vi "Close.vi"(8 "error in":errorcluster, 11 "Comport":refnum<visa-resource-name>) -> (0 "error out":errorcluster)   [LabVIEW 2020, in "MicroPythonClient.lvlib"]
doc: "Closes the comport to the target"
uses:
  MicroPythonClient.lvlib
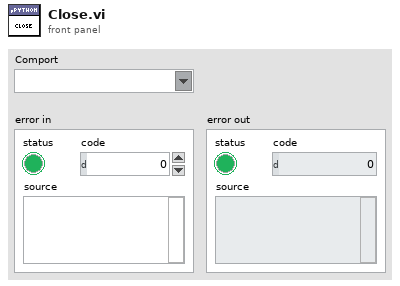
[diagram p1: front panel]
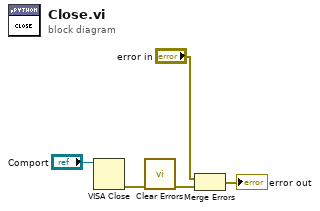
[diagram p0: block diagram]
diagram:
  n1 = VISA Close(VISA resource name="Comport") -> (error out=w2:errorcluster)  [unwired: 1 in]
  n2 = call <vilib>:"Clear Errors.vi"("error in (no error)"=w2) -> ("error out"=w1:errorcluster)  [unwired: 5 in, 1 out]
  n3 = Merge Errors("error in", w1) -> (→"error out":errorcluster)
